vi "画像データポインタでの画像操作呼び出し.vi"() -> ()   [LabVIEW 2020]
uses:
  <vilib>/vision/NI_Vision_Development_Module.lvlib
  DLL/VisionImageManipulationTest1/Debug/VisionImageManipulationTest1.dll
panel:
  out "x - y":u32
  out "Image 2":T1(plugin-control)
  in  "停止":bool
  out "Image":T1(plugin-control)
  # "俺のPCで１回あたり約0.12ms\nCorei5-6200U"
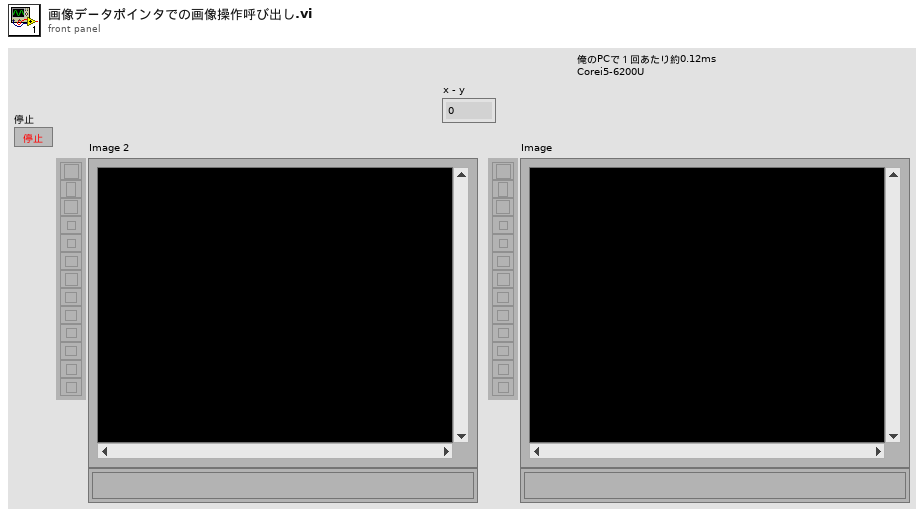
[diagram p1: front panel]
types:
  T1 = typedef "IMAQ Image.ctl" = refnum<image>
  T2 = typedef "Image Type" = u32
  T3 = enum32{"Map Pixel Pointer", "Unmap Pixel Pointer", "Get Pixels Infos"}
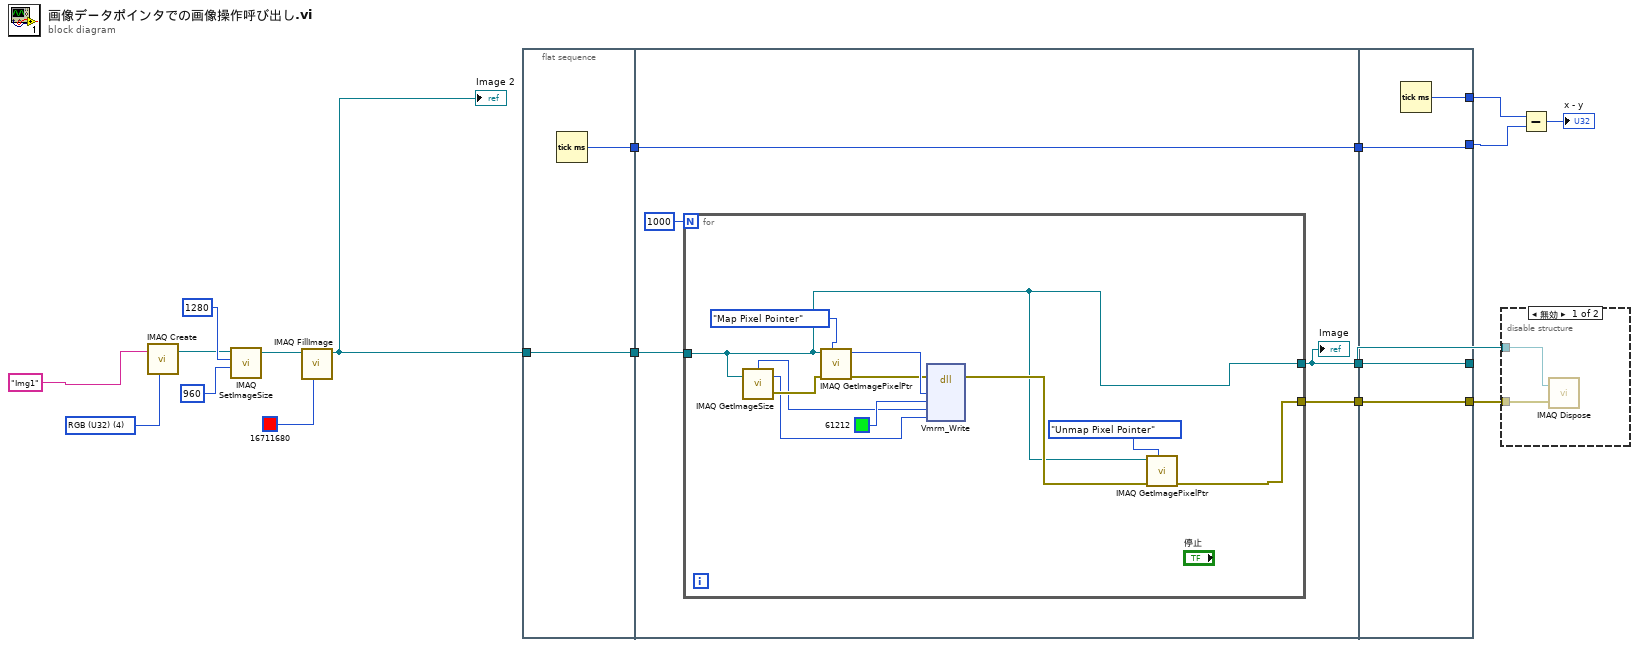
[diagram p0: block diagram]
diagram:
  w10 = T2 4 items=["Grayscale (U8)", "Grayscale (I16)", "Grayscale (SGL)", "Complex (CSG)", "RGB (U32)", "HSL (U32)", "RGB (U64)", "Grayscale (U16)"] ("Image Type")
  n1 = call "IMAQ Create"("Image Name"="Img1" ("形式文字列"), "Image Type"=w10) -> ("New Image"=w14:T1)  [unwired: 3 in, 1 out]
  n2 = call "IMAQ SetImageSize"("Y Resolution"=960, "X Resolution"=1280, "Image"=w14) -> ("Image Out"=w17:T1)  [unwired: 2 in, 1 out]
  n3 = call "IMAQ FillImage"("Color Pixel Value"=u32 16711680, "Image"=w17) -> ("Image Out"=w11:T1)  [unwired: 8 in, 1 out]
  "Image 2" <- w11
  n4 = flat-sequence {
    tunnel: w11 -> [w20]
    tunnel: [w20] -> w8
    tunnel: [w19] -> w5
    tunnel: w8 -> [w24]
    tunnel: [w25] -> w7
    tunnel: [w21] -> w6
    tunnel: w5 -> [w23]
    tunnel: [w23] -> w4
    tunnel: [w39] -> w9
    tunnel: [w40] -> w13
    tunnel: w7 -> [w40]
    tunnel: w6 -> [w39]
    tunnel: w4 -> [w38]
    tunnel: [w38] -> w2
    tunnel: [w37] -> w3
    frame #0 {
      n5 = Tick Count (ms)() -> (millisecond timer value=w19:u32)
    }
    frame #1 {
      n6 = for {
        N: 1000 -> [_]
        tunnel: [w30] -> w25
        tunnel: w24 -> [w29]
        tunnel: [w29] -> w21
        n7 = call "IMAQ GetImageSize"("Image"=w29) -> ("Y Resolution"=w26:i32, "X Resolution"=w27:i32, "error out"=w28:errorcluster)  [unwired: 3 in]
        n8 = call "IMAQ GetImagePixelPtr"("Function"=T3."Map Pixel Pointer", "error in (no error)"=w28, "Image"=w29) -> ("error out"=w35:errorcluster, "Pixel Pointer out"=w36:u64)  [unwired: 3 in, 4 out]
        n9 = dll-call lib="PTH2abs CUserskasaiDesktop(IMAQã®ãã¼ã¿ç´æ¥æä½ã«ã¤ãã¦å®é¨VIDLLVisionImageManipulationTest1Debug VisionImageManipulationTest1.dll" fn="Vmrm_Write"(error in=w35, "vmem"=w36, "color"=u32 61212, "xsize"=w27, "ysize"=w26) -> (error out=w31:errorcluster)  [unwired: 7 in, 1 out]
        n10 = call "IMAQ GetImagePixelPtr"("Function"=T3."Unmap Pixel Pointer", "error in (no error)"=w31, "Image"=w29) -> ("error out"=w30:errorcluster)  [unwired: 3 in, 5 out]
      }
      "Image" <- w21
    }
    frame #2 {
      n11 = Tick Count (ms)() -> (millisecond timer value=w37:u32)
    }
  }
  n12 = disable-structure shown="無効" {
    disable-tunnel: w13 -> [w42 _]
    disable-tunnel: w9 -> [w41 _]
    frame Disabled {
      n13 = call "IMAQ Dispose"("Image"=w41, "error in (no error)"=w42) -> ()  [unwired: 4 in, 1 out]
    }
    frame Enabled {
    }
  }
  n14 = Subtract(x=w3, y=w2) -> (x-y=→"x - y":u32)
